vi "multiplier to index converter.vi"(4 "Multiplier":T1) -> (1 "Index":dbl)   [LabVIEW 2018]
uses:
  Multiplier--control.ctl
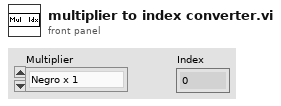
[diagram p1: front panel]
types:
  T1 = typedef "Multiplier--control.ctl" = enum16{"Negro x 1", "Marron x 10", "Rojo x 100", "Naranja x 1K", "Amarillo x 10K", "Verde x 100K", " Azul x 1M", "Violeta x 10M ", "Oro x 0.1", "Plata x 0.01"}
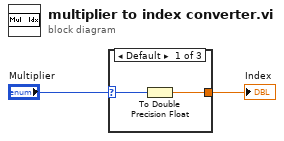
[diagram p0: block diagram]
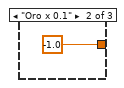
[diagram p2: hidden frame]
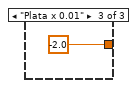
[diagram p3: hidden frame]
diagram:
  n1 = case shown="Default" "Multiplier" {
    selector: "Multiplier" -> [w4 _ _]
    tunnel: [w3 -1.0 -2.0] -> w1
    frame Default {
      n2 = To Double Precision Float(number=w4) -> (double precision float=w3:dbl)
    }
    frame "Oro x 0.1" {
    }
    frame "Plata x 0.01" {
    }
  }
  "Index" <- w1
